vi "occMapPathPlanner.vi"() -> ()   [LabVIEW 2018]
uses:
  <vilib>/Model Interface Toolkit/Model Interface Toolkit.lvclass/Model Interface Toolkit.ctl
  <vilib>/Model Interface Toolkit/Model Update.vi
  <vilib>/Model Interface Toolkit/Tick Model.vi
  <vilib>/Model Interface Toolkit/Probe Signals.vi
  <vilib>/Model Interface Toolkit/Multirate/Dispatch Model Tasks.vi
  <vilib>/Model Interface Toolkit/Call Model Start Routine.vi
  <vilib>/Model Interface Toolkit/Handle Error.vi
  <vilib>/Model Interface Toolkit/Multirate/Wait on Tasks.vi
  GlobalVariables.vi
  <vilib>/addons/control/pid/pid.llb/PID (DBL).vi
  <vilib>/Model Interface Toolkit/Check Error.vi
  <vilib>/Model Interface Toolkit/Generate Error Cluster.vi
  <vilib>/Platform/TimedLoop/scheduler/LVUserAPI/Fire Software-Triggered Timing Source.vi
  <vilib>/Model Interface Toolkit/Model Interface Toolkit.lvclass
  <vilib>/addons/control/pid/NI_PID_pid.lvlib
panel:
  out "offset":dbl(graph)
  out "scatterPointOffset":dbl(graph)
  out "yaw":dbl
  out "scatterPointOffset":sgl
  out "vehLoXYS":dbl[](array[numeric])
  out "Hz control":dbl
  in  "P lv":dbl=70.0
  in  "I lv":dbl
  in  "D lv":dbl=0.01
  out "steerAngle lv":dbl
  out "offset":dbl
  in  "preDist":dbl=7.0
  in  "I":dbl
  in  "D":dbl=0.3
  in  "P":dbl=46.0
  out "steerAngle":dbl
  out "isTraNotOK":sgl
  out "xysVehBest":sgl[](array[numeric])
  out "xysCartBest":sgl[](array[numeric])
  in  "occMapCollisionEnable":bool=TRUE
  in  "traCollisionEnable":bool
  in  "missionFlag":u8=1
  out "Hz planning":dbl
  out "路径":path
  out "lon":dbl format="%#.11g"
  out "lat":dbl format="%#.11g"
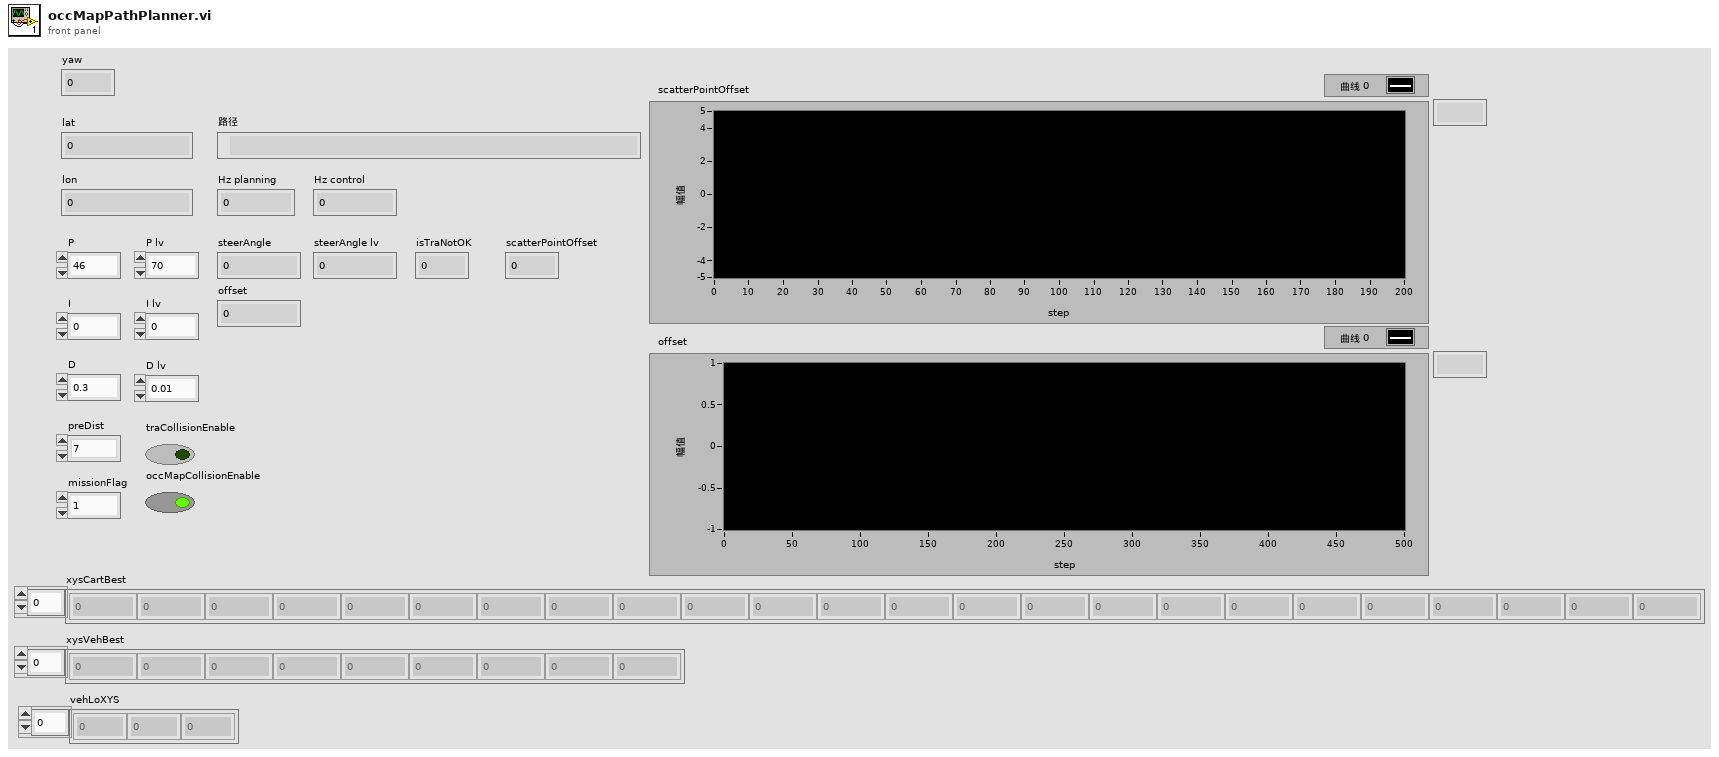
[diagram p1: front panel]
types:
  T1 = cluster{"EMS+ECS+EPS Enable":bool, "HAD_Angle_Wheel":dbl, "HAD_Anglular_Velocity":dbl}
  T2 = cluster{"Name":string, "port":string, "sequence":string, "idleTime":string, "timeStatus":string, "week":string, "seconds":string, "receiverStatus":string, "reserved":string, "receiverVersion":string, "insStatus":string, "posType":string, "lat":string, "lon":string, "height":string, "undulation":string, "northVel":string, "eastVel":string, "upVel":string, "roll":string, "pitch":string, "azimuth":string, "latStandardDevivation":string, "lonStandardDevivation":string, "heightStandardDevivation":string, "northStandardDevivation":string, "eastStandardDevivation":string, "upStandardDevivation":string, "rollStandardDevivation":string, "pitchStandardDevivation":string, "azimuthStandardDevivation":string, "extSolSat":string, "timeSinceUpdate":string, "CRC":string, "#INSPVAXA":string}
  T3 = cluster{"angle":sgl[], "range":sgl[], "intensity":sgl[], "xVeh":sgl[], "yVeh":sgl[], "zVeh":sgl[], "xCart":sgl[], "yCart":sgl[]}
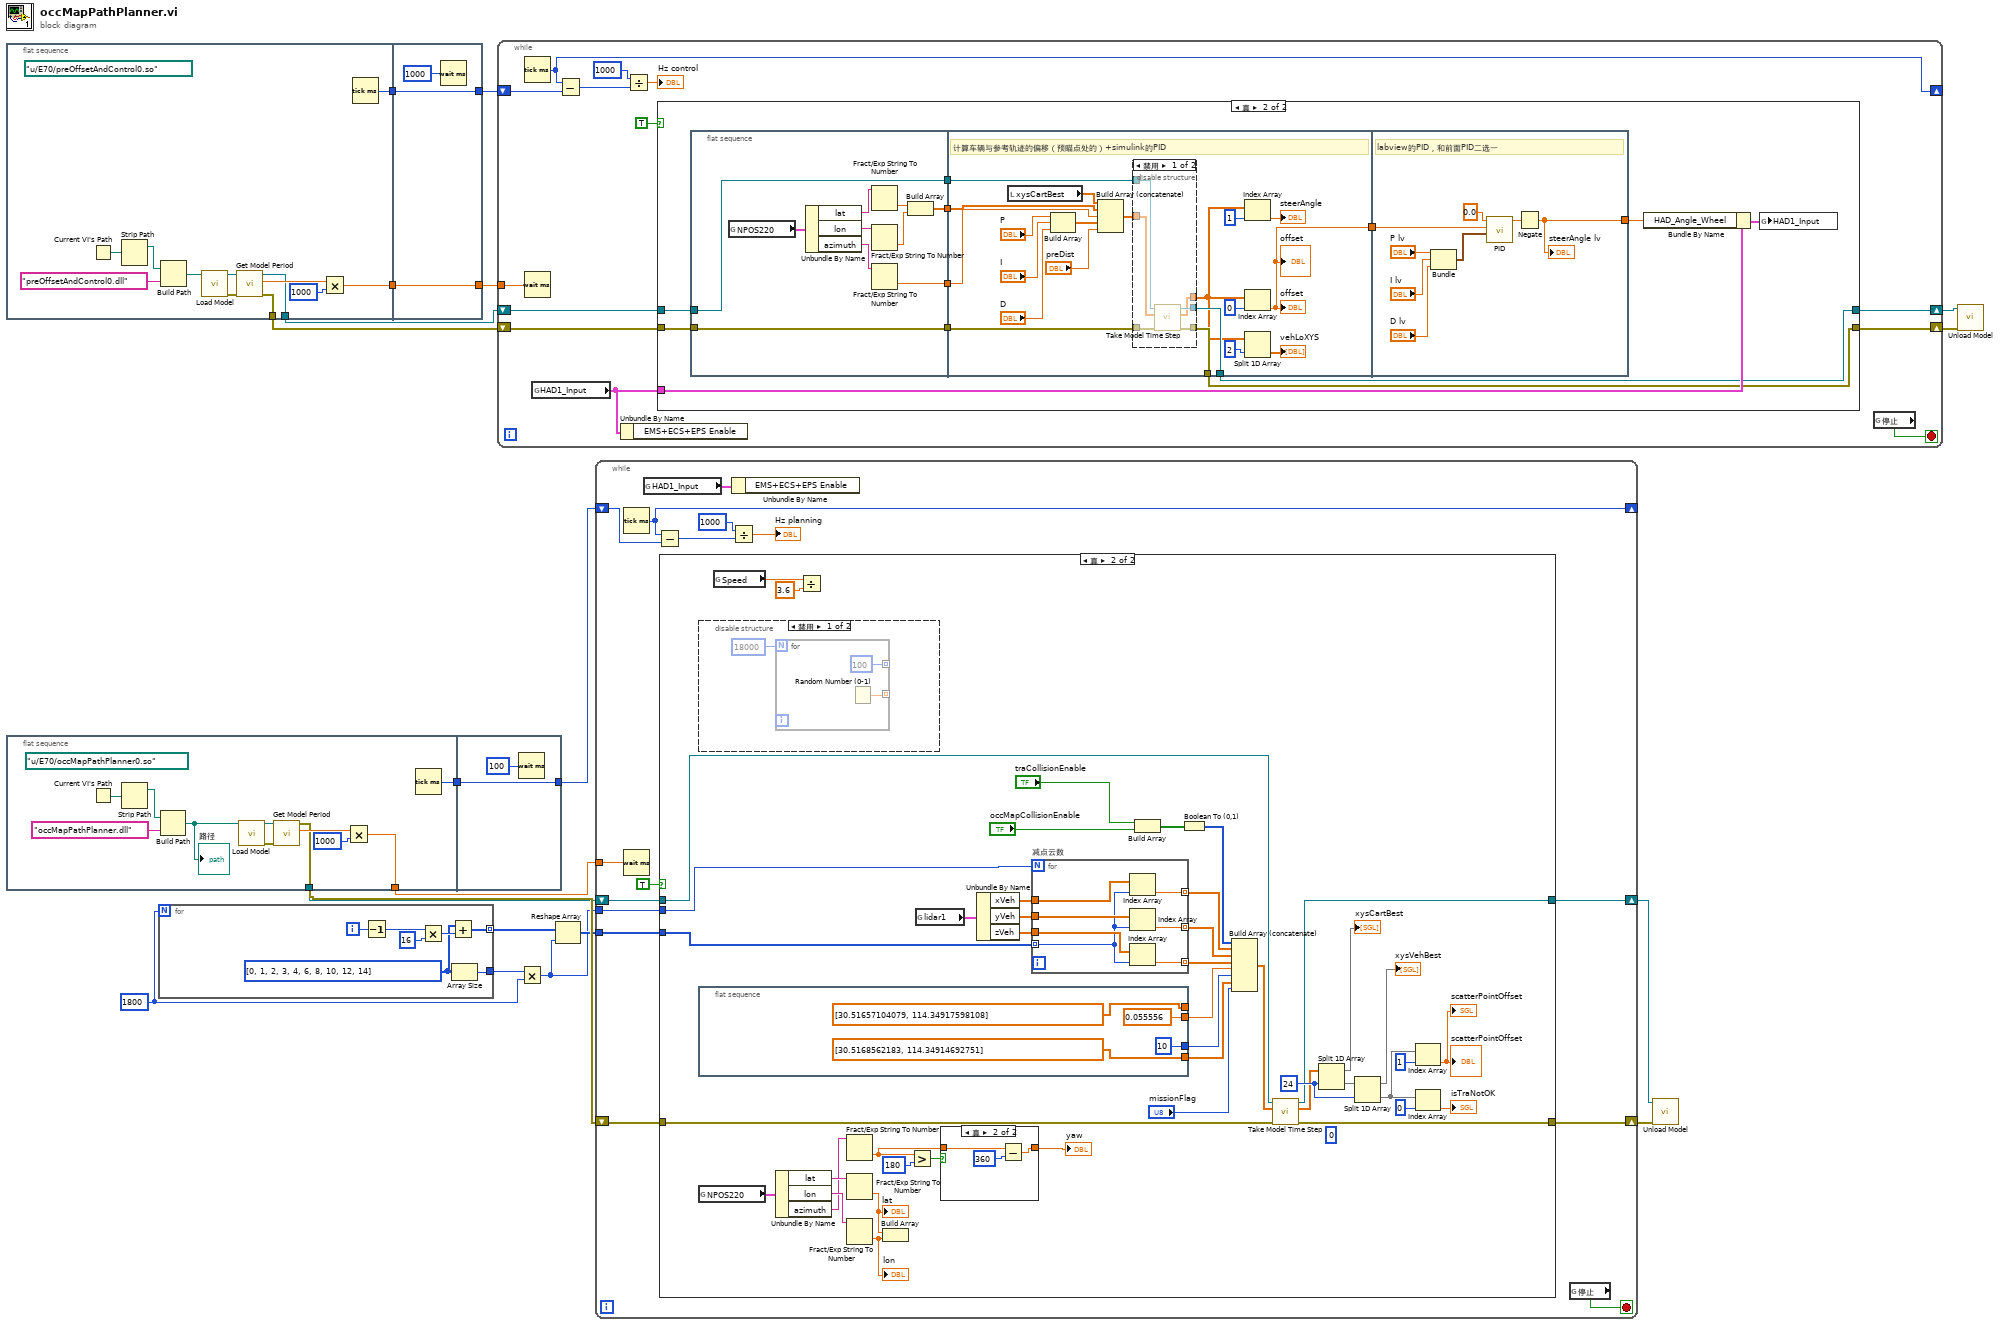
[diagram p0: block diagram]
diagram:
  w4 = 1800
  n1 = flat-sequence {
    tunnel: [w32] -> w12
    tunnel: [w31] -> w11
    tunnel: [w23] -> w9
    tunnel: [w22] -> w8
    tunnel: [w34] -> w13
    tunnel: [w35] -> w19
    tunnel: w12 -> [w35]
    tunnel: w11 -> [w34]
    frame #0 {
      (unwired) path "u:/E70/preOffsetAndControl0.so"
      n2 = Current VI's Path() -> (path=w26:path)
      n3 = Strip Path(path=w26) -> (stripped path=w27:path)  [unwired: 1 out]
      n4 = Build Path(base path=w27, name or relative path="preOffsetAndControl0.dll") -> (appended path=w21:path)
      n5 = call <vilib>:"Load Model.vi"("Model Path"=w21) -> ("error out"=w30:errorcluster, "Model out"=w29:refnum<class "Model Interface Toolkit.lvclass">)  [unwired: 9 in]
      n6 = call <vilib>:"Get Model Period.vi"("error in"=w30, "Model in"=w29) -> ("error out"=w22:errorcluster, "Model Period (s)"=w28:dbl, "Model out"=w23:refnum<class "Model Interface Toolkit.lvclass">)  [unwired: 7 in]
      n7 = Multiply(x=w28, y=1000) -> (x*y=w31:dbl)
      n8 = Tick Count (ms)() -> (millisecond timer value=w32:u32)
    }
    frame #1 {
      n9 = Wait (ms)(milliseconds to wait=1000) -> ()  [unwired: 1 out]
    }
  }
  n10 = flat-sequence {
    tunnel: [w46] -> w14
    tunnel: [w47] -> w10
    tunnel: [w38] -> w7
    tunnel: [w37] -> w6
    tunnel: [w49] -> w20
    tunnel: w10 -> [w49]
    frame #0 {
      (unwired) path "u:/E70/occMapPathPlanner0.so"
      n11 = Current VI's Path() -> (path=w42:path)
      n12 = Strip Path(path=w42) -> (stripped path=w41:path)  [unwired: 1 out]
      n13 = Build Path(base path=w41, name or relative path="occMapPathPlanner.dll") -> (appended path=w36:path)
      "路径" <- w36
      n14 = call <vilib>:"Load Model.vi"("Model Path"=w36) -> ("error out"=w39:errorcluster, "Model out"=w40:refnum<class "Model Interface Toolkit.lvclass">)  [unwired: 9 in]
      n15 = call <vilib>:"Get Model Period.vi"("error in"=w39, "Model in"=w40) -> ("error out"=w38:errorcluster, "Model Period (s)"=w44:dbl, "Model out"=w37:refnum<class "Model Interface Toolkit.lvclass">)  [unwired: 7 in]
      n16 = Multiply(x=w44, y=1000) -> (x*y=w46:dbl)
      n17 = Tick Count (ms)() -> (millisecond timer value=w47:u32)
    }
    frame #1 {
      n18 = Wait (ms)(milliseconds to wait=100) -> ()  [unwired: 1 out]
    }
  }
  n19 = for {
    N: w4 -> [_]
    tunnel: [w51] -> w5
    tunnel: [w50] -> w3 mode=indexing
    i -> [w56]
    w52 = i32[] [0, 1, 2, 3, 4, 6, 8, 10, 12, 14]
    n20 = Decrement(x=w56) -> (x-1=w54:i32)
    n21 = Multiply(x=w54, y=16) -> (x*y=w53:i32)
    n22 = Add(x=w52, y=w53) -> (x+y=w50:i32[])
    n23 = Array Size(array=w52) -> (size(s)=w51:i32)
  }
  n24 = while {
    shift-right: [w64] -> _
    shift-left: w19 -> [w67]
    shift-right: [w59] -> w18
    shift-left: w9 -> [w61]
    shift-right: [w60] -> w17
    shift-left: w8 -> [w62]
    tunnel: w13 -> [w58]
    stop <- w69 stop-if-true
    n25 = Tick Count (ms)() -> (millisecond timer value=w64:u32)
    n26 = Wait (ms)(milliseconds to wait=w58) -> ()  [unwired: 1 out]
    n27 = global read "GlobalVariables.vi" "HAD1_Input"() -> (w63:T1)
    n28 = Subtract(x=w64, y=w67) -> (x-y=w66:u32)
    n29 = Unbundle By Name(w63) -> ()  [unwired: 1 out]
    n30 = Divide(x=1000, y=w66) -> (x/y=→"Hz control":dbl)
    n31 = case shown="真" TRUE {
      tunnel: w63 -> [_ w83]
      tunnel: [w71 w77] -> w60
      tunnel: w62 -> [w71 w79]
      tunnel: w61 -> [w70 w78]
      tunnel: [w70 w74] -> w59
      frame False {
      }
      frame True {
        n32 = flat-sequence "平铺式顺序结构" {
          tunnel: w78 -> [w92]
          tunnel: w79 -> [w93]
          tunnel: [w93] -> w76
          tunnel: [w92] -> w75
          tunnel: [w85] -> w73
          tunnel: [w84] -> w72
          tunnel: [w94] -> w80
          tunnel: [w102] -> w77
          tunnel: w76 -> [w103]
          tunnel: w75 -> [w105]
          tunnel: [w101] -> w74
          tunnel: w73 -> [w96]
          tunnel: w72 -> [w95]
          tunnel: [w120] -> w81
          tunnel: w80 -> [w122]
          frame #0 {
            n33 = global read "GlobalVariables.vi" "NPOS220"() -> (w88:T2)
            n34 = Unbundle By Name(w88) -> ("lat"=w90:string, "lon"=w89:string, "azimuth"=w91:string)
            n35 = Fract/Exp String To Number(string=w90) -> (number=w87:dbl)  [unwired: 3 in, 1 out]
            n36 = Fract/Exp String To Number(string=w89) -> (number=w86:dbl)  [unwired: 3 in, 1 out]
            n37 = Fract/Exp String To Number(string=w91) -> (number=w84:dbl)  [unwired: 3 in, 1 out]
            n38 = Build Array(w87, w86) -> (w85:dbl[])
          }
          frame #1 {
            # "计算车辆与参考轨迹的偏移（预瞄点处的）+simulink的PID"
            n39 = local read "xysCartBest"() -> (w100:sgl[])
            n40 = Build Array("P", "I", "D") -> (w110:dbl[])
            n41 = Build Array (concatenate)(w100, w96, w95, w110, "preDist") -> (w104:dbl[])
            n42 = disable-structure shown="禁用" {
              disable-tunnel: w105 -> [w119 _]
              disable-tunnel: w104 -> [w118 _]
              disable-tunnel: w103 -> [w117 _]
              disable-tunnel: [w116 _] -> w102
              disable-tunnel: [w115 _] -> w101
              disable-tunnel: [w114 _] -> w99
              frame Disabled {
                n43 = call <vilib>:"Take Model Time Step.vi"("error in (no error)"=w117, "Inport Array"=w118, "Model in"=w119) -> ("error out"=w116:errorcluster, "Outport Array out"=w114:dbl[], "Model out"=w115:refnum<class "Model Interface Toolkit.lvclass">)  [unwired: 6 in]
              }
              frame Enabled {
              }
            }
            n44 = Index Array(array=w99, index=1) -> (element=→"steerAngle":dbl)
            n45 = Index Array(array=w99, index=0) -> (element=w94:dbl)
            "offset" <- w94
            "offset" <- w94
            n46 = Split 1D Array(array=w99, index=2) -> (second subarray=→"vehLoXYS":dbl[])  [unwired: 1 out]
          }
          frame #2 {
            # "labview的PID，和前面PID二选一"
            n47 = Bundle("P lv"="P lv", "I lv"="I lv", "D lv"="D lv") -> (w124:cluster{"P lv":dbl, "I lv":dbl, "D lv":dbl})  [unwired: 1 in]
            n48 = call-poly <vilib>:"PID.vi"("PID gains"=w124, "process variable"=w122, "setpoint"=0.0) -> ("output"=w121:dbl)  [unwired: 7 in, 1 out]
            n49 = Negate(x=w121) -> (-x=w120:dbl)
            "steerAngle lv" <- w120
          }
        }
        n50 = Bundle By Name(cluster=w83, "HAD_Angle_Wheel"=w81) -> (w82:T1)
        n51 = global write "GlobalVariables.vi" "HAD1_Input"(w82) -> ()
      }
    }
    n52 = global read "GlobalVariables.vi" "停止"() -> (w69:bool)
  }
  n53 = Multiply(x=w5, y=w4) -> (x*y=w1:i32)
  n54 = Reshape Array(w3, w1) -> (w2:i32[])
  n55 = while {
    shift-right: [w136] -> _
    shift-left: w20 -> [w135]
    shift-right: [w133] -> w16
    shift-left: w6 -> [w140]
    shift-right: [w134] -> w15
    shift-left: w7 -> [w141]
    tunnel: w14 -> [w132]
    tunnel: w1 -> [w129]
    tunnel: w2 -> [w128]
    stop <- w142 stop-if-true
    n56 = Tick Count (ms)() -> (millisecond timer value=w136:u32)
    n57 = Wait (ms)(milliseconds to wait=w132) -> ()  [unwired: 1 out]
    n58 = global read "GlobalVariables.vi" "HAD1_Input"() -> (w131:T1)
    n59 = Subtract(x=w136, y=w135) -> (x-y=w138:u32)
    n60 = case shown="真" TRUE {
      tunnel: w141 -> [w144 w186]
      tunnel: w140 -> [w143 w187]
      tunnel: [w144 w185] -> w134
      tunnel: [w143 w172] -> w133
      tunnel: w129 -> [_ w150]
      tunnel: w128 -> [_ w149]
      frame False {
      }
      frame True {
        (unwired) 0
        w183 = 24
        n61 = disable-structure shown="禁用" {
          frame Disabled {
            n62 = for {
              N: 18000 -> [_]
              tunnel: [w195] -> _ mode=indexing
              tunnel: [100] -> _ mode=indexing
              n63 = Random Number (0-1)() -> (number: 0 to 1=w195:dbl)
            }
          }
          frame Enabled {
          }
        }
        n64 = flat-sequence {
          tunnel: [dbl[] [30.51657104079, 114.34917598108]] -> _
          tunnel: [10] -> w147
          tunnel: [dbl[] [30.5168562183, 114.34914692751]] -> w146
          tunnel: [0.055556] -> w148
          frame #0 {
          }
        }
        n65 = global read "GlobalVariables.vi" "NPOS220"() -> (w160:T2)
        n66 = global read "GlobalVariables.vi" "Speed"() -> (w158:dbl)
        n67 = Unbundle By Name(w160) -> ("lat"=w163:string, "lon"=w162:string, "azimuth"=w161:string)
        n68 = Divide(x=w158, y=3.6) -> ()  [unwired: 1 out]
        n69 = Fract/Exp String To Number(string=w161) -> (number=w152:dbl)  [unwired: 3 in, 1 out]
        n70 = Fract/Exp String To Number(string=w163) -> (number=w164:dbl)  [unwired: 3 in, 1 out]
        "lat" <- w164
        n71 = Fract/Exp String To Number(string=w162) -> (number=w165:dbl)  [unwired: 3 in, 1 out]
        "lon" <- w165
        n72 = Build Array(w164, w165) -> ()  [unwired: 1 out]
        n73 = Greater?(x=w152, y=180) -> (0:w153:bool)
        n74 = global read "GlobalVariables.vi" "lidar1"() -> (w166:T3)
        n75 = case shown="真" w153 {
          tunnel: w152 -> [w189 w191]
          tunnel: [w189 w190] -> w151
          frame False {
          }
          frame True {
            n76 = Subtract(x=w191, y=360) -> (x-y=w190:dbl)
          }
        }
        "yaw" <- w151
        n77 = Unbundle By Name(w166) -> ("xVeh"=w169:sgl[], "yVeh"=w168:sgl[], "zVeh"=w167:sgl[])
        n78 = for "减点云数" {
          N: w150 -> [_]
          tunnel: w168 -> [w206]
          tunnel: w167 -> [w205]
          tunnel: w169 -> [w204]
          tunnel: [w203] -> w156 mode=indexing
          tunnel: [w201] -> w155 mode=indexing
          tunnel: [w202] -> w157 mode=indexing
          tunnel: w149 -> [w200] mode=indexing
          n79 = Index Array(array=w204, index=w200) -> (element=w202:sgl)
          n80 = Index Array(array=w206, index=w200) -> (element=w201:sgl)
          n81 = Index Array(array=w205, index=w200) -> (element=w203:sgl)
        }
        n82 = Build Array("traCollisionEnable", "occMapCollisionEnable") -> (w173:bool[])
        n83 = Boolean To (0,1)(Boolean=w173) -> (0, 1=w176:i16[])
        n84 = Build Array (concatenate)(w176, w157, w155, w156, w148, w147, w146, "missionFlag") -> (w184:dbl[])
        n85 = call <vilib>:"Take Model Time Step.vi"("error in (no error)"=w186, "Inport Array"=w184, "Model in"=w187) -> ("error out"=w185:errorcluster, "Outport Array out"=w180:dbl[], "Model out"=w172:refnum<class "Model Interface Toolkit.lvclass">)  [unwired: 6 in]
        n86 = Split 1D Array(array=w180, index=w183) -> (first subarray=→"xysCartBest":dbl[], second subarray=w182:dbl[])
        n87 = Split 1D Array(array=w182, index=w183) -> (first subarray=→"xysVehBest":dbl[], second subarray=w170:dbl[])
        n88 = Index Array(array=w170, index=1) -> (element=→"scatterPointOffset" →"scatterPointOffset":dbl)
        n89 = Index Array(array=w170, index=0) -> (element=→"isTraNotOK":dbl)
      }
    }
    n90 = Divide(x=1000, y=w138) -> (x/y=→"Hz planning":dbl)
    n91 = Unbundle By Name(w131) -> ()  [unwired: 1 out]
    n92 = global read "GlobalVariables.vi" "停止"() -> (w142:bool)
  }
  n93 = call <vilib>:"Unload Model.vi"("error in (no error)"=w15, "Model in"=w16) -> ()  [unwired: 9 in, 1 out]
  n94 = call <vilib>:"Unload Model.vi"("error in (no error)"=w17, "Model in"=w18) -> ()  [unwired: 9 in, 1 out]
